vi "PIV_POD.vi"(0 "Data Folder":path=path "T:/Ensight_Data/NACA0015/NACA0015_NM_B/Test_A", 1 "PIV Meas Plane":enum16{"XY", "YZ", "XZ"}(ring)=enum."XZ", 2 "Row number":i32=1, 5 "Output Directory":path=path "T:/Ensight_Data/NACA0015/NACA0015_NM_B", 7 "XYZ Translation":dbl[](array[numeric])=[200.0, 8.0, -30.0], 9 "Case Name":string="Test_A_Case", 11 "PIV Freq (Hz)":dbl=7.25, 12 "Invert U":bool=TRUE, 13 "Invert V":bool) -> (4 "Progress Bar":i32(slide) scale=0.0..100.0, 6 "Status":string, 10 "# total vectors":i32=9858)   [LabVIEW 2022 SP3]
uses:
  <vilib>/Analysis/NI_AALBase.lvlib
  <vilib>/Analysis/1siggen.llb/Ramp Pattern by Samples.vi
  <vilib>/Utility/error.llb/DialogType.ctl
  <vilib>/Analysis/Matrix/NI_Matrix.lvlib
  <vilib>/Analysis/Matrix/Numeric/Multiply/Multiply - RM,RM.vi
  <vilib>/Analysis/NI_AALPro.lvlib
  <vilib>/Analysis/7linalg.llb/Real Eigenvalues and Vectors.vi
  <vilib>/Analysis/Matrix/Numeric/Conversions/Matrix To Array - CM.vi
  <vilib>/Analysis/Matrix/Numeric/Conversions/Array To Matrix - RA.vi
  <vilib>/Analysis/Matrix/Numeric/Conversions/Matrix To Array - RM.vi
  <vilib>/Analysis/Matrix/Numeric/Conversions/Array To Matrix - RA2.vi
panel:
  in  "Spot Data Cluster":T1
  out "u(Spot,mode)":dbl[][](array[numeric])
  out "v(Spot,mode)":dbl[][](array[numeric])
  out "Modal Energy":dbl[](array[numeric])
  out "eVal":dbl[](array[numeric]) format="%.2f"
  out "eVec":dbl[][](array[numeric])
  out "Uall(Spot,time)":dbl[][](array[numeric])
  out "v'(Spot,time)":dbl[][](array[numeric])
  out "u'(Spot,time)":dbl[][](array[numeric])
  out "Data Array (spot,Var)":dbl[][](array[numeric])
  out "File Paths":path[](array[path])
  out "Position Array (XYZ,spot)":dbl[][](array[numeric])
  out "Variable Names":string[](array[string])=["Record_Length", "CHC", "u_ms", "v_ms", "time_s", "Vel_mag_ms", "Turb_Stats_U_ms", "Turb_Stats_u2_m2s2", "Turb_Stats_u3_m3s3", "Turb_Stats_u4_m4s4", "Turb_Stats_TurbU_%", "Turb_Stats_Skew_u", "Turb_Stats_Kurt_u", "Turb_Stats_V_ms", "Turb_Stats_v2_m2s2", "Turb_Stats_v3_m3s3", "Turb_Stats_v4_m4s4", "Turb_Stats_TurbV_%", "Turb_Stats_Skew_v", "Turb_Stats_Kurt_v", "Turb_Stats_u2v2_m4s4", "Turb_Stats_uv3_m4s4", "Turb_Stats_u3v_m4s4", "Turb_Stats_uv2_m3s3", "Turb_Stats_u2v_m3s3", "Turb_Stats_uv_cc", "Turb_Stats_uv", "Turb_Stats_TKE_J", "Turb_Stats_Error_U_ms", "Turb_Stats_Error_u2_m2s2", "Turb_Stats_Error_u3_m3s3", "Turb_Stats_Error_u4_m4s4", "Turb_Stats_Error_TurbU_%", "Turb_Stats_Error_Skew_u", "Turb_Stats_Error_Kurt_u", "Turb_Stats_Error_V_ms", "Turb_Stats_Error_v2_m2s2", "Turb_Stats_Error_v3_m3s3", "Turb_Stats_Error_v4_m4s4", "Turb_Stats_Error_TurbV_%", "Turb_Stats_Error_Skew_v", "Turb_Stats_Error_Kurt_v", "Turb_Stats_Error_u2v2_m4s4", "Turb_Stats_Error_uv3_m4s4", "Turb_Stats_Error_u3v_m4s4", "Turb_Stats_Error_uv2_m3s3", "Turb_Stats_Error_u2v_m3s3", "Turb_Stats_Error_uv_cc", "Turb_Stats_Error_uv", "Turb_Stats_Error_TKE_J"]
  out "time s":dbl[](array[numeric])=[0.0, 0.20689655172413793, 0.41379310344827586]
  out "File Array":path[](array[path])=[path "T:/Ensight_Data/NACA0015/NACA0015_NM_A/Test_A_Trans/New folder/Test_A000000.T076.D000.P000.H000.L.vec", path "T:/Ensight_Data/NACA0015/NACA0015_NM_A/Test_A_Trans/New folder/Test_A000001.T076.D000.P000.H000.L.vec", path "T:/Ensight_Data/NACA0015/NACA0015_NM_A/Test_A_Trans/New folder/Test_A000002.T076.D000.P000.H000.L.vec"]
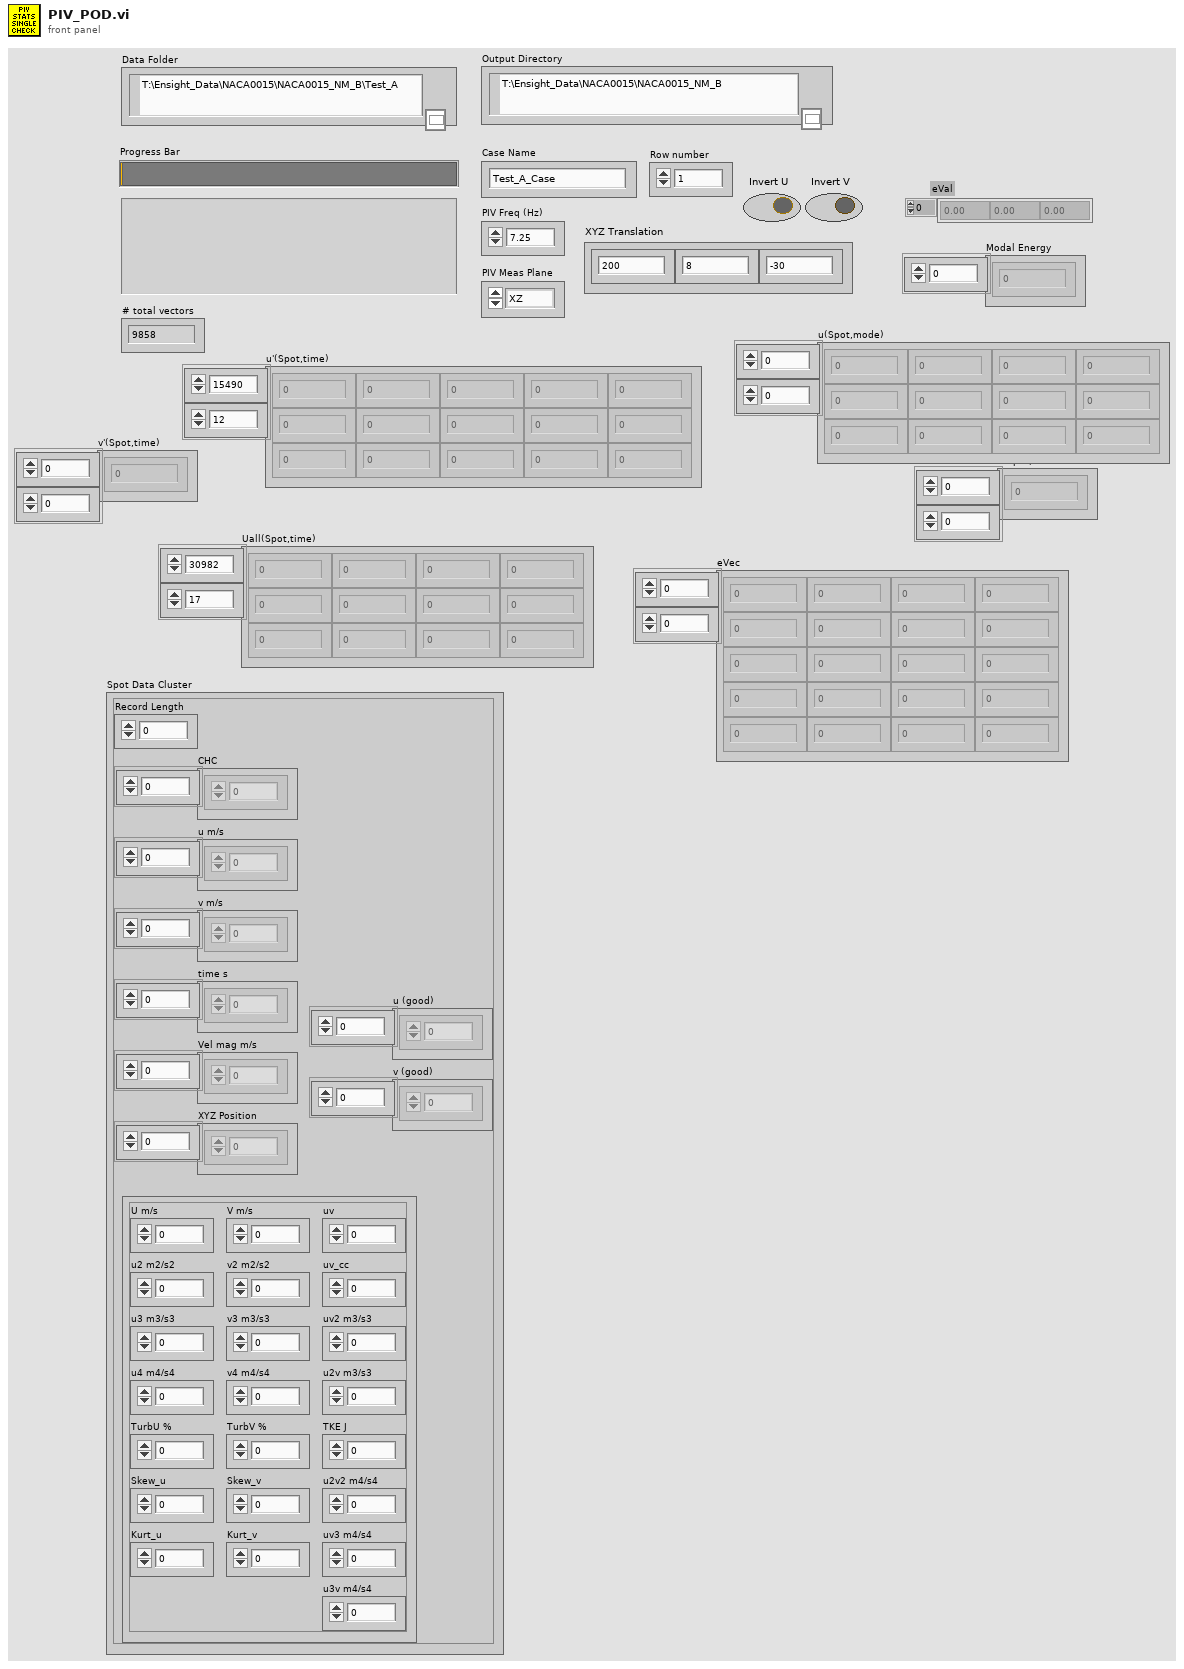
[diagram p1: front panel]
types:
  T1 = cluster{"Record Length":dbl, "CHC":dbl[], "u m/s":dbl[], "v m/s":dbl[], "time s":dbl[], "Vel mag m/s":dbl[], "XYZ Position":dbl[], "Turbulence Statistics":cluster{"U m/s":dbl, "u2 m2/s2":dbl, "u3 m3/s3":dbl, "u4 m4/s4":dbl, "TurbU %":dbl, "Skew_u":dbl, "Kurt_u":dbl, "V m/s":dbl, "v2 m2/s2":dbl, "v3 m3/s3":dbl, "v4 m4/s4":dbl, "TurbV %":dbl, "Skew_v":dbl, "Kurt_v":dbl, "u2v2 m4/s4":dbl, "uv3 m4/s4":dbl, "u3v m4/s4":dbl, "uv2 m3/s3":dbl, "u2v m3/s3":dbl, "uv_cc":dbl, "uv":dbl, "TKE J":dbl}, "v (good)":dbl[], "u (good)":dbl[]}
  T2 = cluster{"Record Length":dbl, "CHC":dbl[], "u m/s":dbl[], "v m/s":dbl[], "time s":dbl[], "Vel mag m/s":dbl[], "XYZ Position":dbl[], "Turbulence Statistics":cluster{"U m/s":dbl, "u2 m2/s2":dbl, "u3 m3/s3":dbl, "u4 m4/s4":dbl, "TurbU %":dbl, "Skew_u":dbl, "Kurt_u":dbl, "V m/s":dbl, "v2 m2/s2":dbl, "v3 m3/s3":dbl, "v4 m4/s4":dbl, "TurbV %":dbl, "Skew_v":dbl, "Kurt_v":dbl, "u2v2 m4/s4":dbl, "uv3 m4/s4":dbl, "u3v m4/s4":dbl, "uv2 m3/s3":dbl, "u2v m3/s3":dbl, "uv_cc":dbl, "uv":dbl, "TKE J":dbl}, "v (good)":dbl[], "u (good)":dbl[]}[]
  T3 = cluster{"Record Length":dbl, "CHC":dbl[], "u m/s":dbl[], "v m/s":dbl[], "time s":dbl[], "Vel mag m/s":dbl[], "XYZ Position":dbl[], " Turb Stats":cluster{"U m/s":dbl, "u2 m2/s2":dbl, "u3 m3/s3":dbl, "u4 m4/s4":dbl, "TurbU %":dbl, "Skew_u":dbl, "Kurt_u":dbl, "V m/s":dbl, "v2 m2/s2":dbl, "v3 m3/s3":dbl, "v4 m4/s4":dbl, "TurbV %":dbl, "Skew_v":dbl, "Kurt_v":dbl, "u2v2 m4/s4":dbl, "uv3 m4/s4":dbl, "u3v m4/s4":dbl, "uv2 m3/s3":dbl, "u2v m3/s3":dbl, "uv_cc":dbl, "uv":dbl, "TKE J":dbl}[], "Turb Stats Error":cluster{"U m/s":dbl, "u2 m2/s2":dbl, "u3 m3/s3":dbl, "u4 m4/s4":dbl, "TurbU %":dbl, "Skew_u":dbl, "Kurt_u":dbl, "V m/s":dbl, "v2 m2/s2":dbl, "v3 m3/s3":dbl, "v4 m4/s4":dbl, "TurbV %":dbl, "Skew_v":dbl, "Kurt_v":dbl, "u2v2 m4/s4":dbl, "uv3 m4/s4":dbl, "u3v m4/s4":dbl, "uv2 m3/s3":dbl, "u2v m3/s3":dbl, "uv_cc":dbl, "uv":dbl, "TKE J":dbl}[], "u (good)":dbl[], "v (good)":dbl[]}
  T4 = cluster{"U m/s":dbl, "u2 m2/s2":dbl, "u3 m3/s3":dbl, "u4 m4/s4":dbl, "TurbU %":dbl, "Skew_u":dbl, "Kurt_u":dbl, "V m/s":dbl, "v2 m2/s2":dbl, "v3 m3/s3":dbl, "v4 m4/s4":dbl, "TurbV %":dbl, "Skew_v":dbl, "Kurt_v":dbl, "u2v2 m4/s4":dbl, "uv3 m4/s4":dbl, "u3v m4/s4":dbl, "uv2 m3/s3":dbl, "u2v m3/s3":dbl, "uv_cc":dbl, "uv":dbl, "TKE J":dbl}
  T5 = cluster{"U m/s":dbl, "u2 m2/s2":dbl, "u3 m3/s3":dbl, "u4 m4/s4":dbl, "TurbU %":dbl, "Skew_u":dbl, "Kurt_u":dbl, "V m/s":dbl, "v2 m2/s2":dbl, "v3 m3/s3":dbl, "v4 m4/s4":dbl, "TurbV %":dbl, "Skew_v":dbl, "Kurt_v":dbl, "u2v2 m4/s4":dbl, "uv3 m4/s4":dbl, "u3v m4/s4":dbl, "uv2 m3/s3":dbl, "u2v m3/s3":dbl, "uv_cc":dbl, "uv":dbl, "TKE J":dbl}[]
  T6 = cluster{"Record Length":dbl, "CHC":dbl[], "u m/s":dbl[], "v m/s":dbl[], "time s":dbl[], "Vel mag m/s":dbl[], "XYZ Position":dbl[], " Turb Stats":cluster{"U m/s":dbl, "u2 m2/s2":dbl, "u3 m3/s3":dbl, "u4 m4/s4":dbl, "TurbU %":dbl, "Skew_u":dbl, "Kurt_u":dbl, "V m/s":dbl, "v2 m2/s2":dbl, "v3 m3/s3":dbl, "v4 m4/s4":dbl, "TurbV %":dbl, "Skew_v":dbl, "Kurt_v":dbl, "u2v2 m4/s4":dbl, "uv3 m4/s4":dbl, "u3v m4/s4":dbl, "uv2 m3/s3":dbl, "u2v m3/s3":dbl, "uv_cc":dbl, "uv":dbl, "TKE J":dbl}[], "Turb Stats Error":cluster{"U m/s":dbl, "u2 m2/s2":dbl, "u3 m3/s3":dbl, "u4 m4/s4":dbl, "TurbU %":dbl, "Skew_u":dbl, "Kurt_u":dbl, "V m/s":dbl, "v2 m2/s2":dbl, "v3 m3/s3":dbl, "v4 m4/s4":dbl, "TurbV %":dbl, "Skew_v":dbl, "Kurt_v":dbl, "u2v2 m4/s4":dbl, "uv3 m4/s4":dbl, "u3v m4/s4":dbl, "uv2 m3/s3":dbl, "u2v m3/s3":dbl, "uv_cc":dbl, "uv":dbl, "TKE J":dbl}[], "u (good)":dbl[], "v (good)":dbl[]}[]
  T7 = typedef "NI_Matrix.lvlib/RealMatrix.ctl" = dbl[][]
  T8 = typedef "NI_Matrix.lvlib/ComplexMatrix.ctl" = cdb[][]
  T9 = typedef "DialogType.ctl" = u16
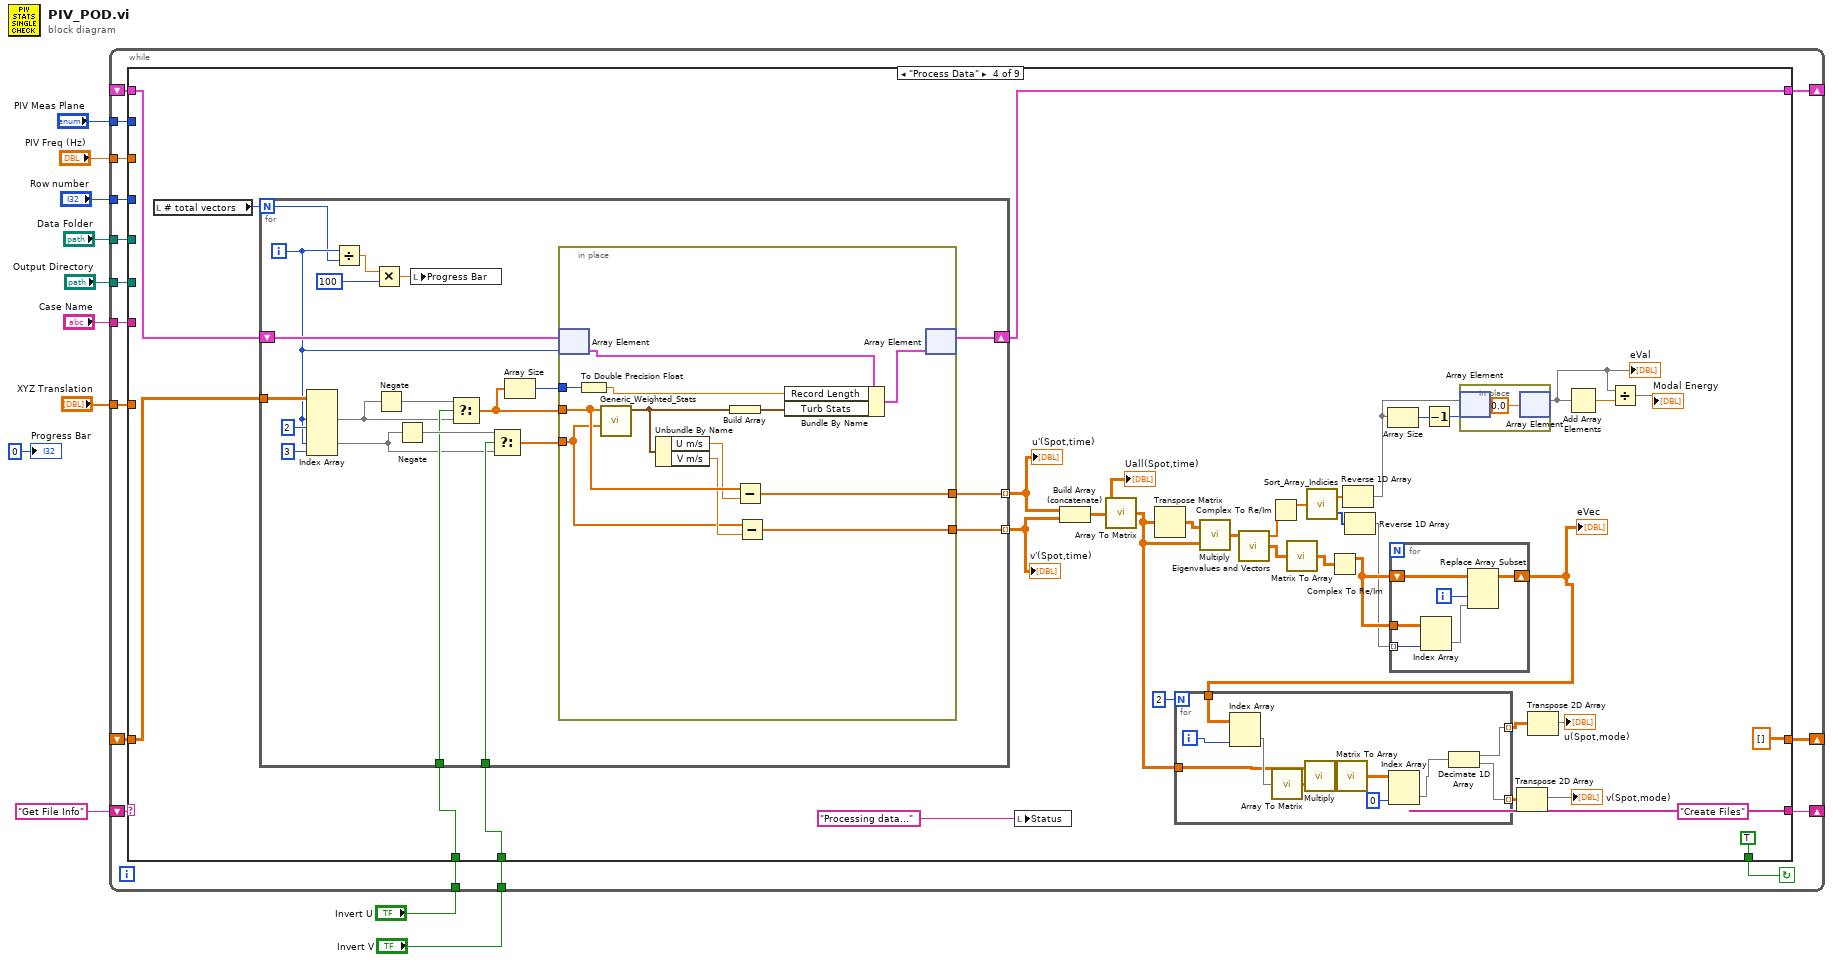
[diagram p0: block diagram]
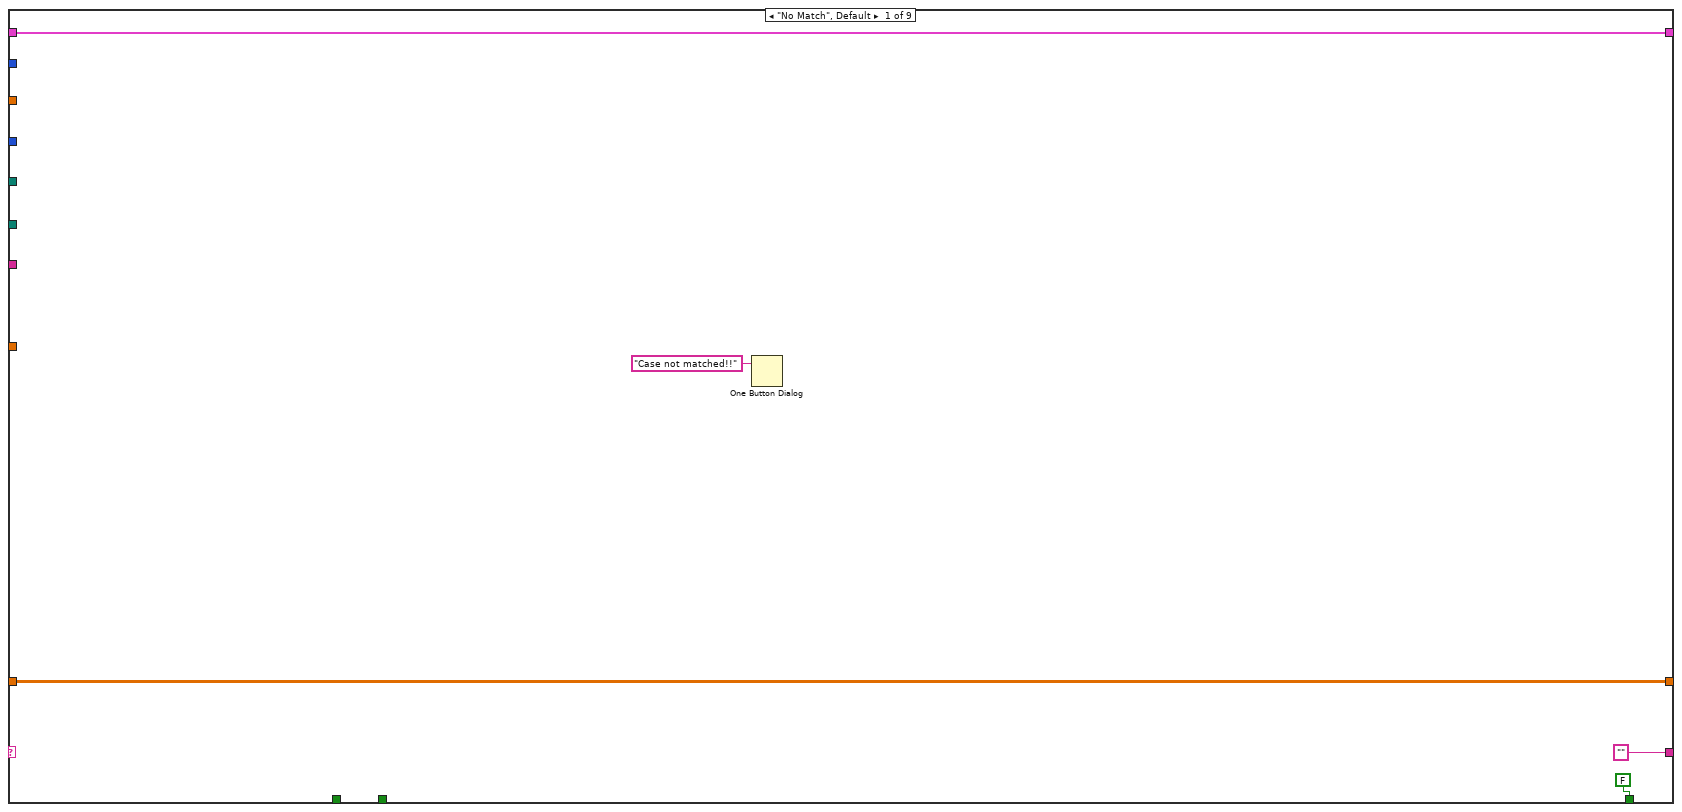
[diagram p2: hidden frame]
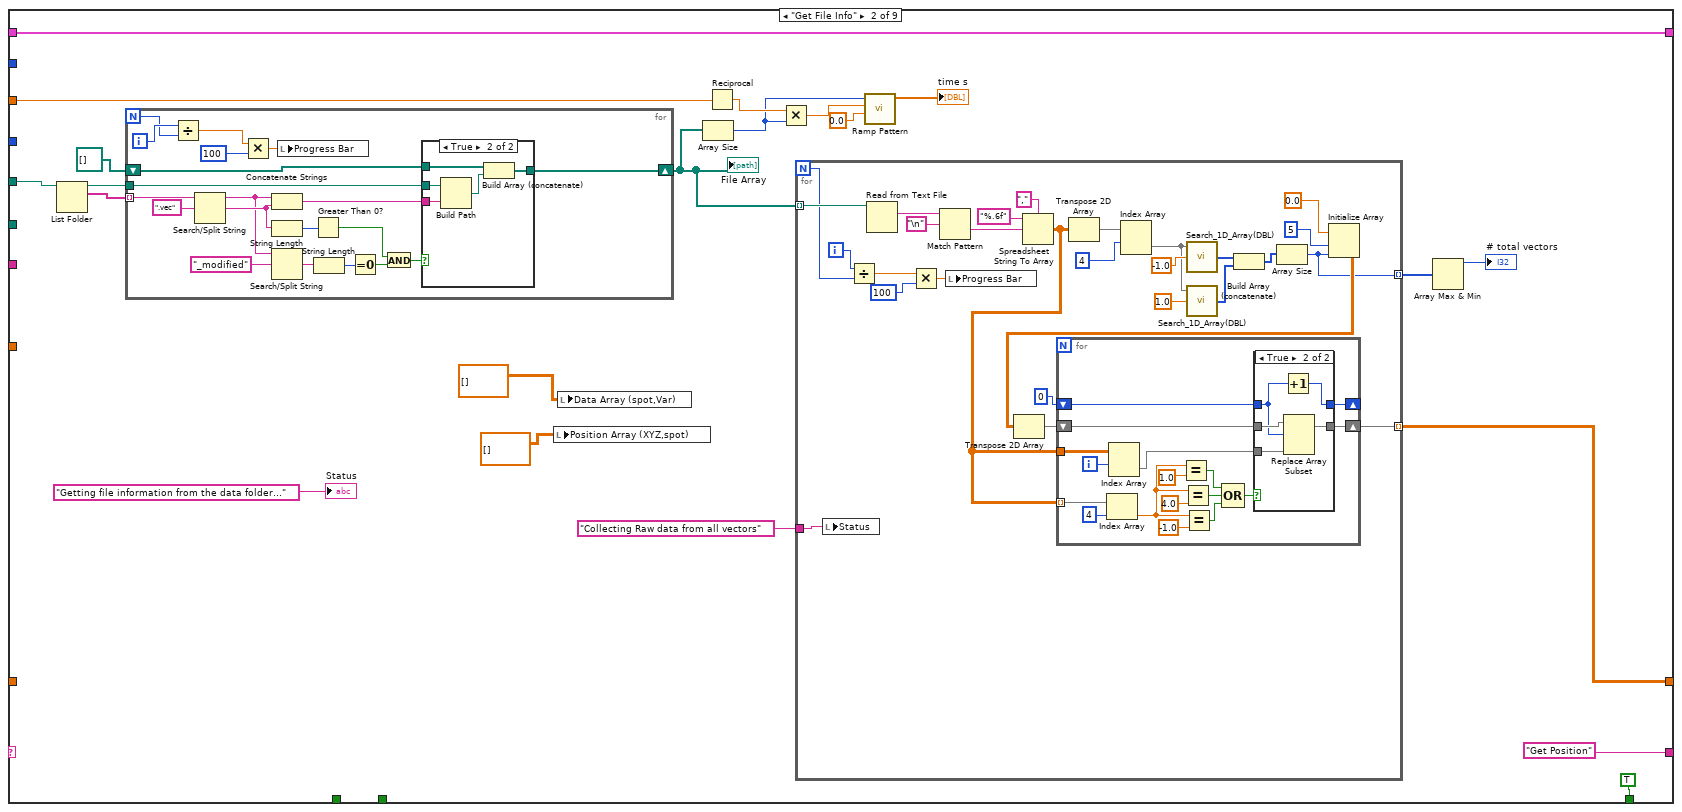
[diagram p3: hidden frame]
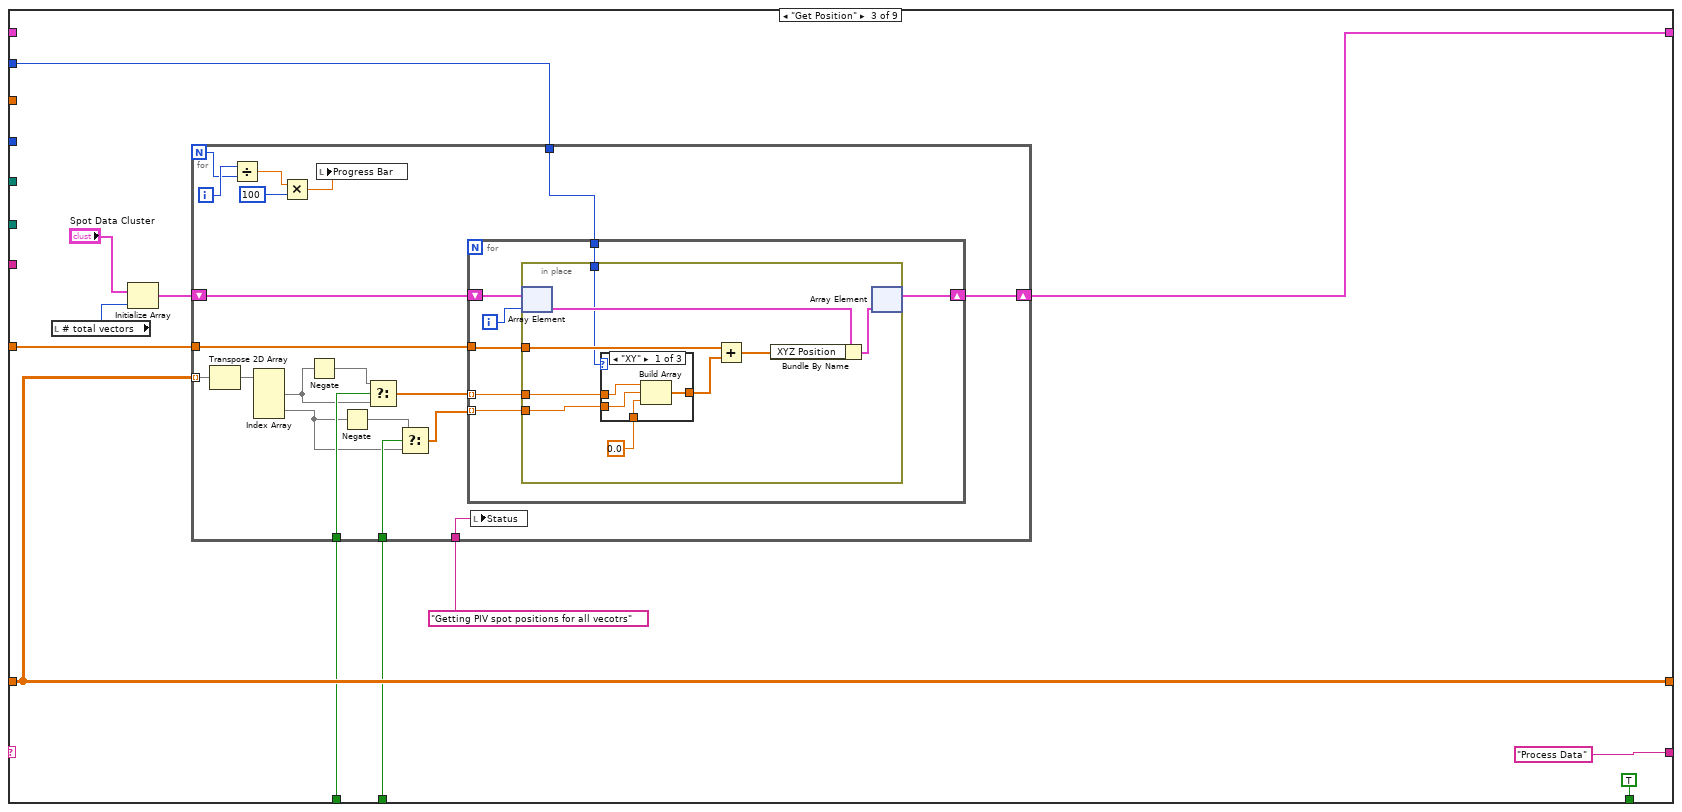
[diagram p6: hidden frame]
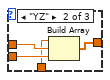
[diagram p7: hidden frame]
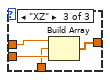
[diagram p8: hidden frame]
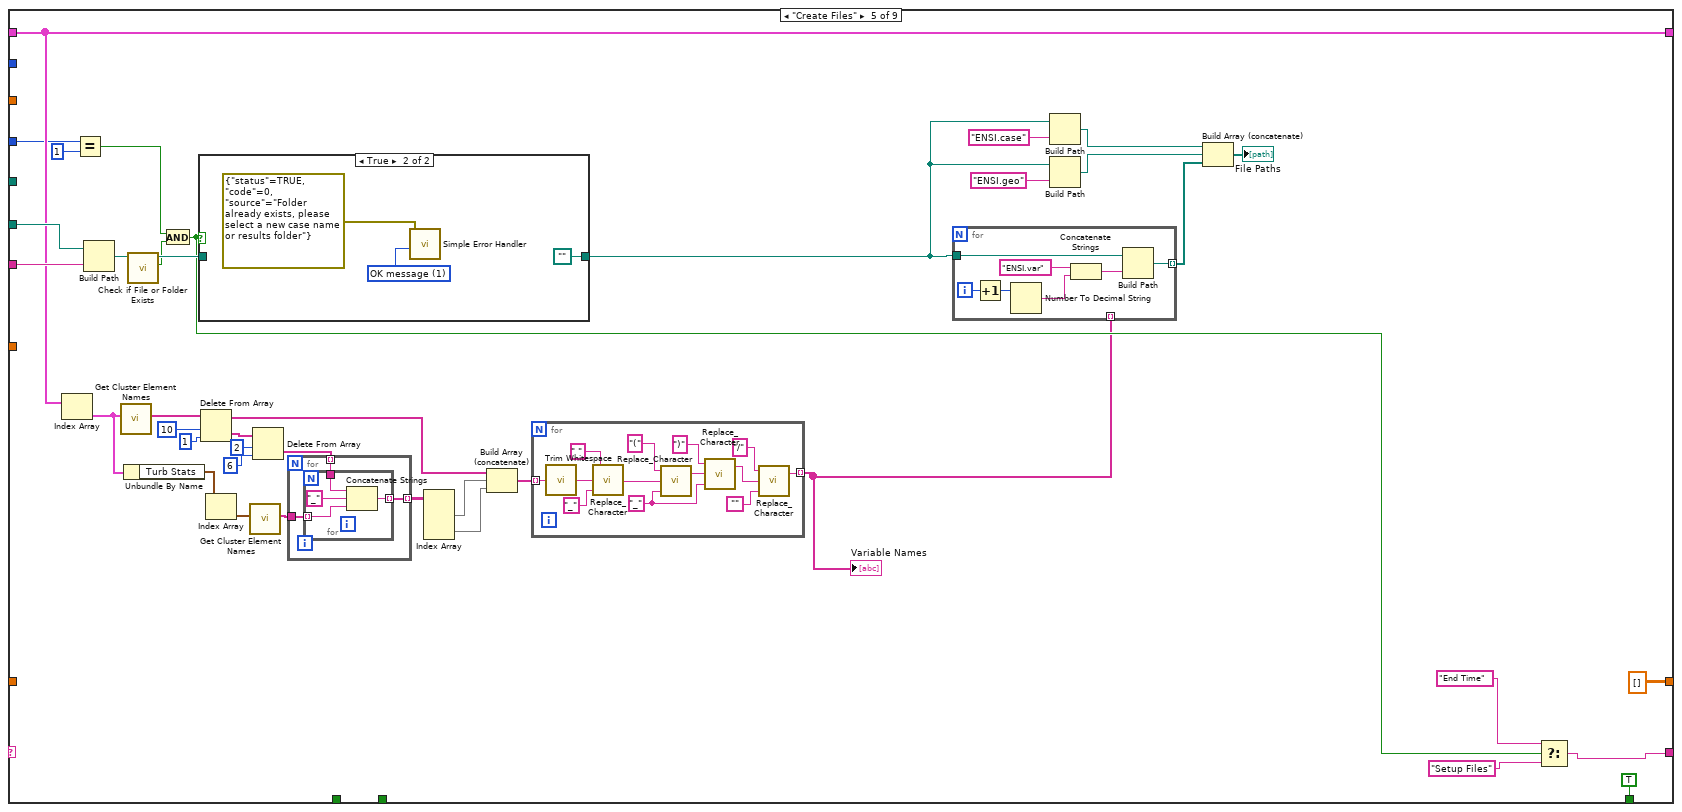
[diagram p9: hidden frame]
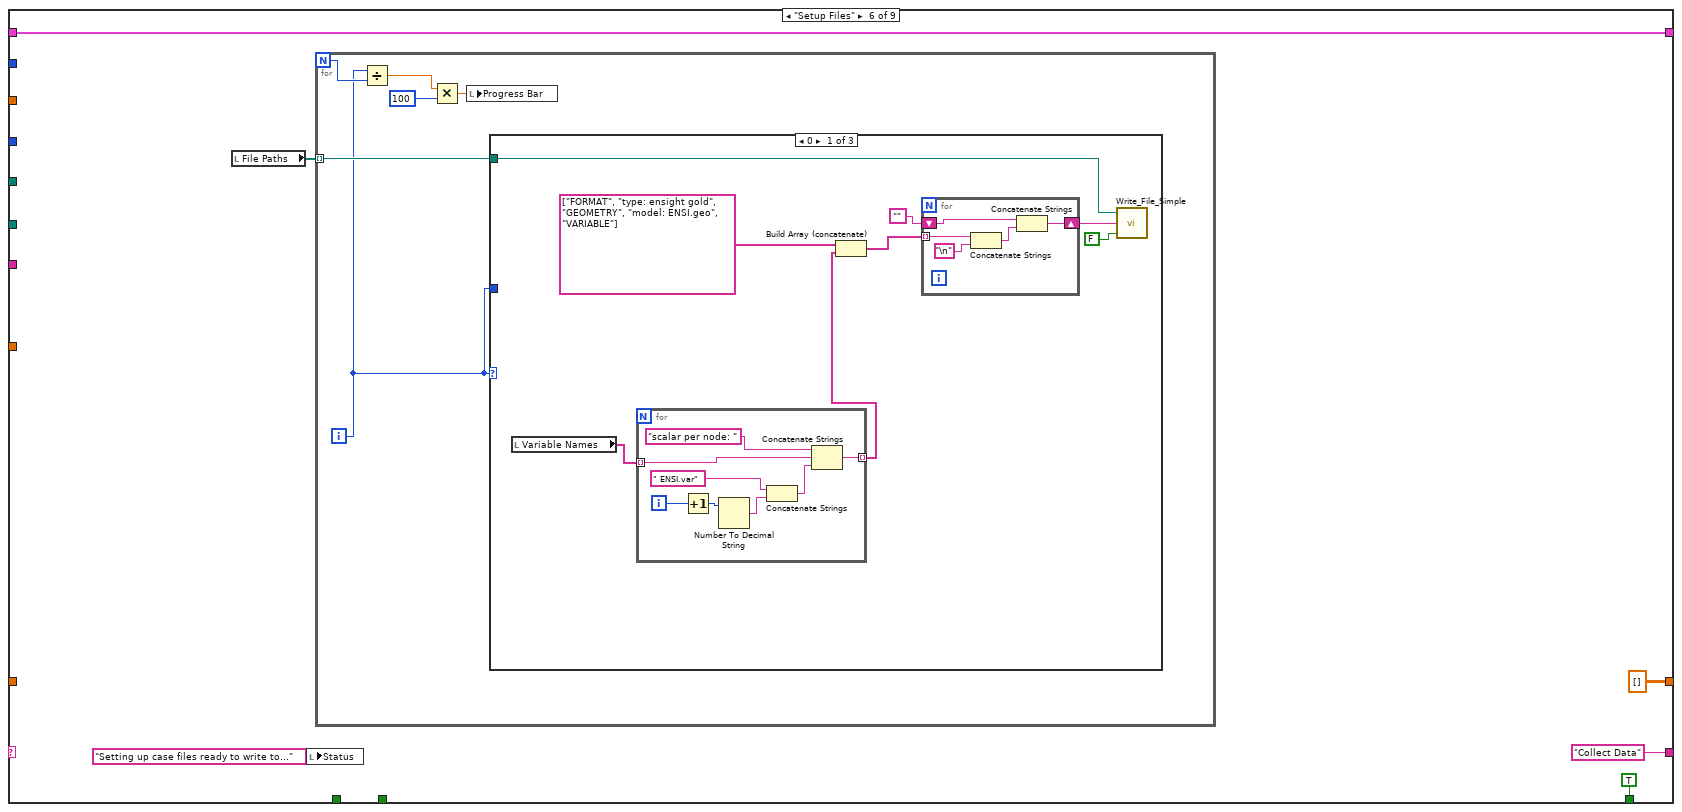
[diagram p11: hidden frame]
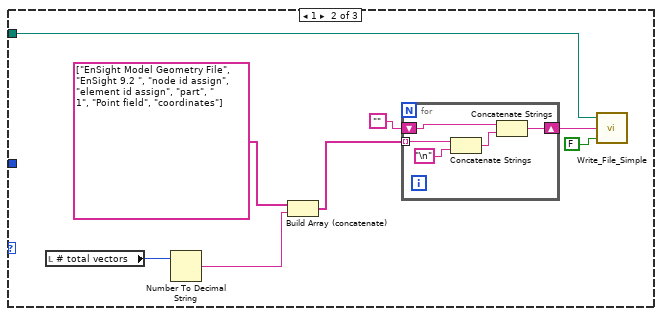
[diagram p12: hidden frame]
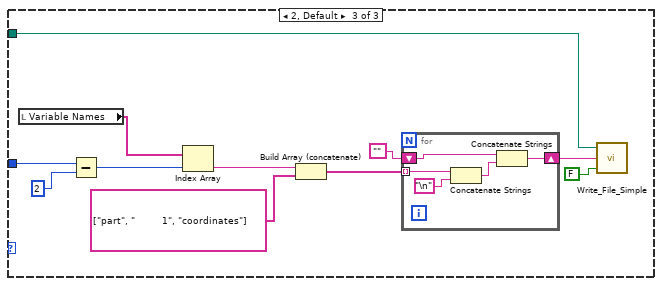
[diagram p13: hidden frame]
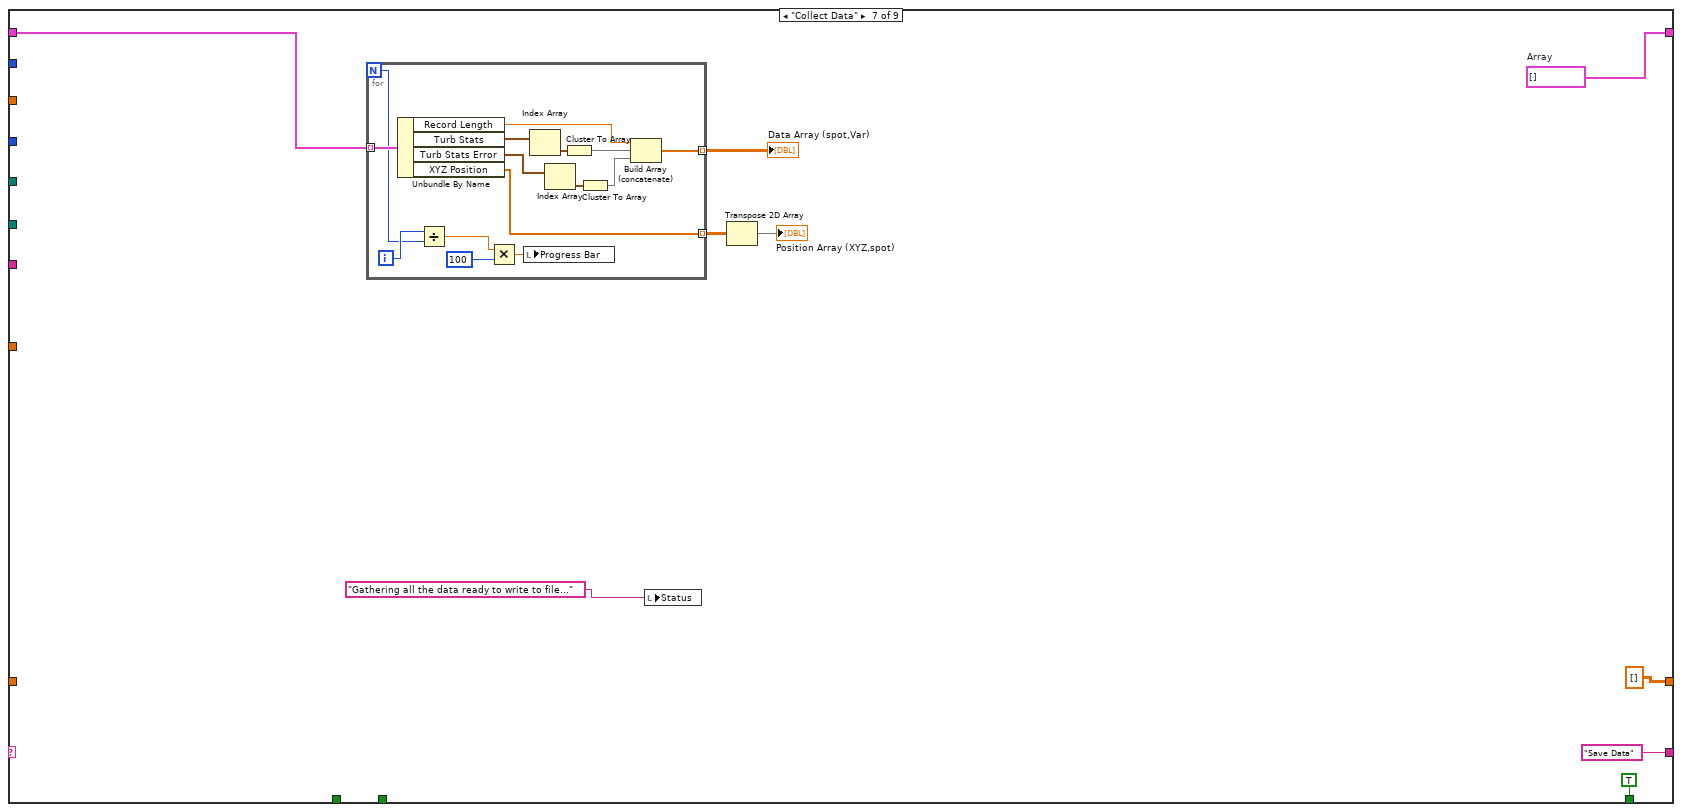
[diagram p14: hidden frame]
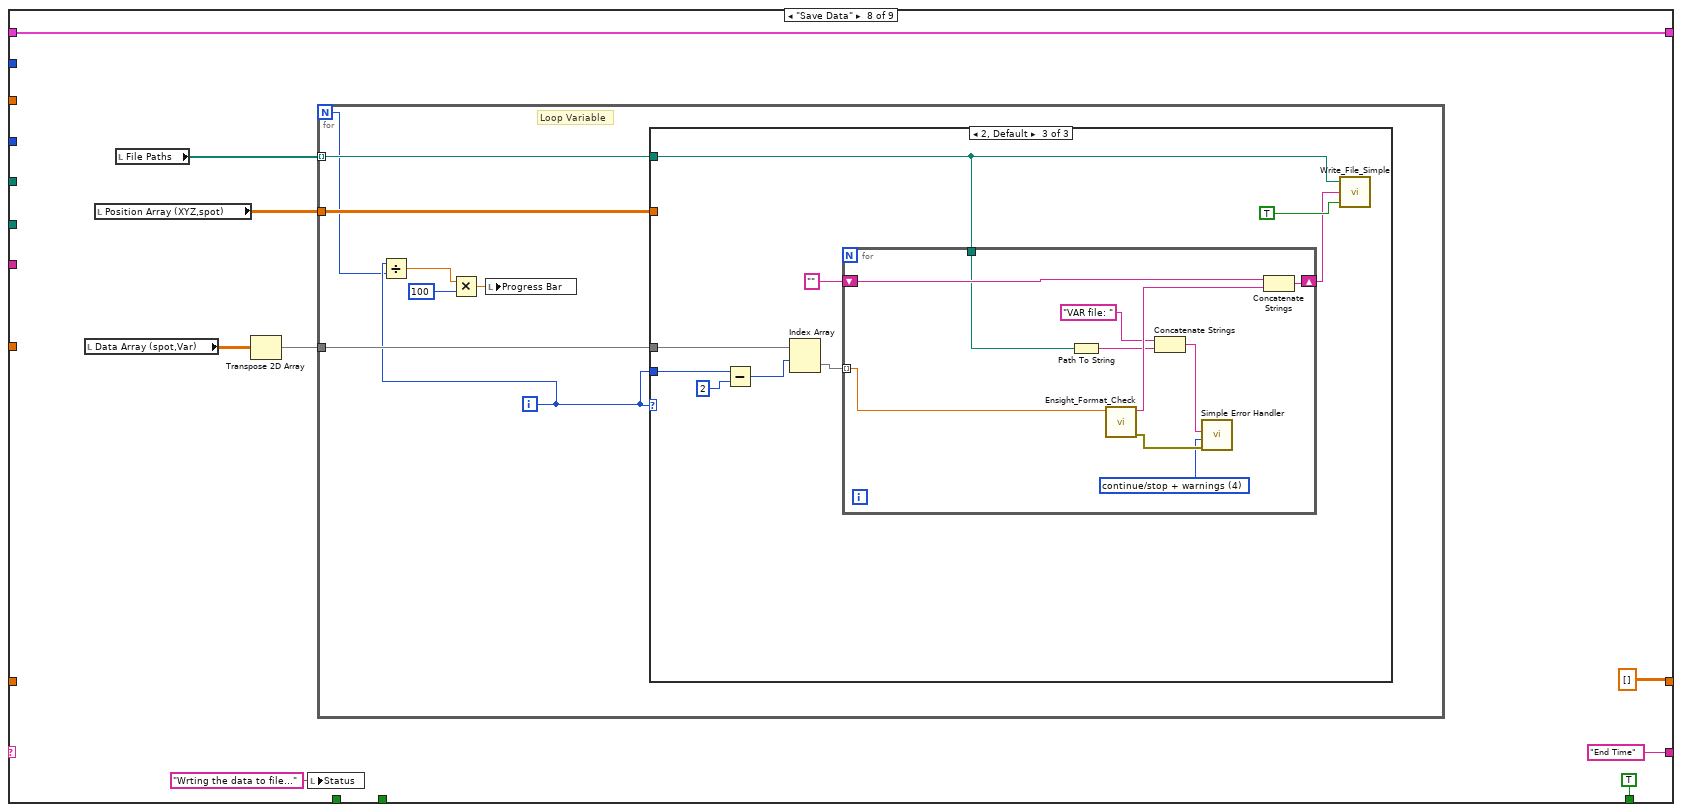
[diagram p15: hidden frame]
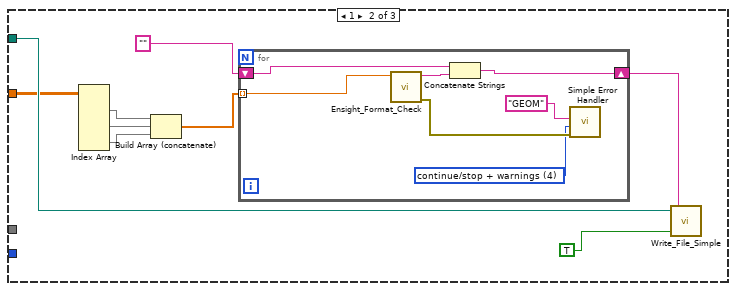
[diagram p17: hidden frame]
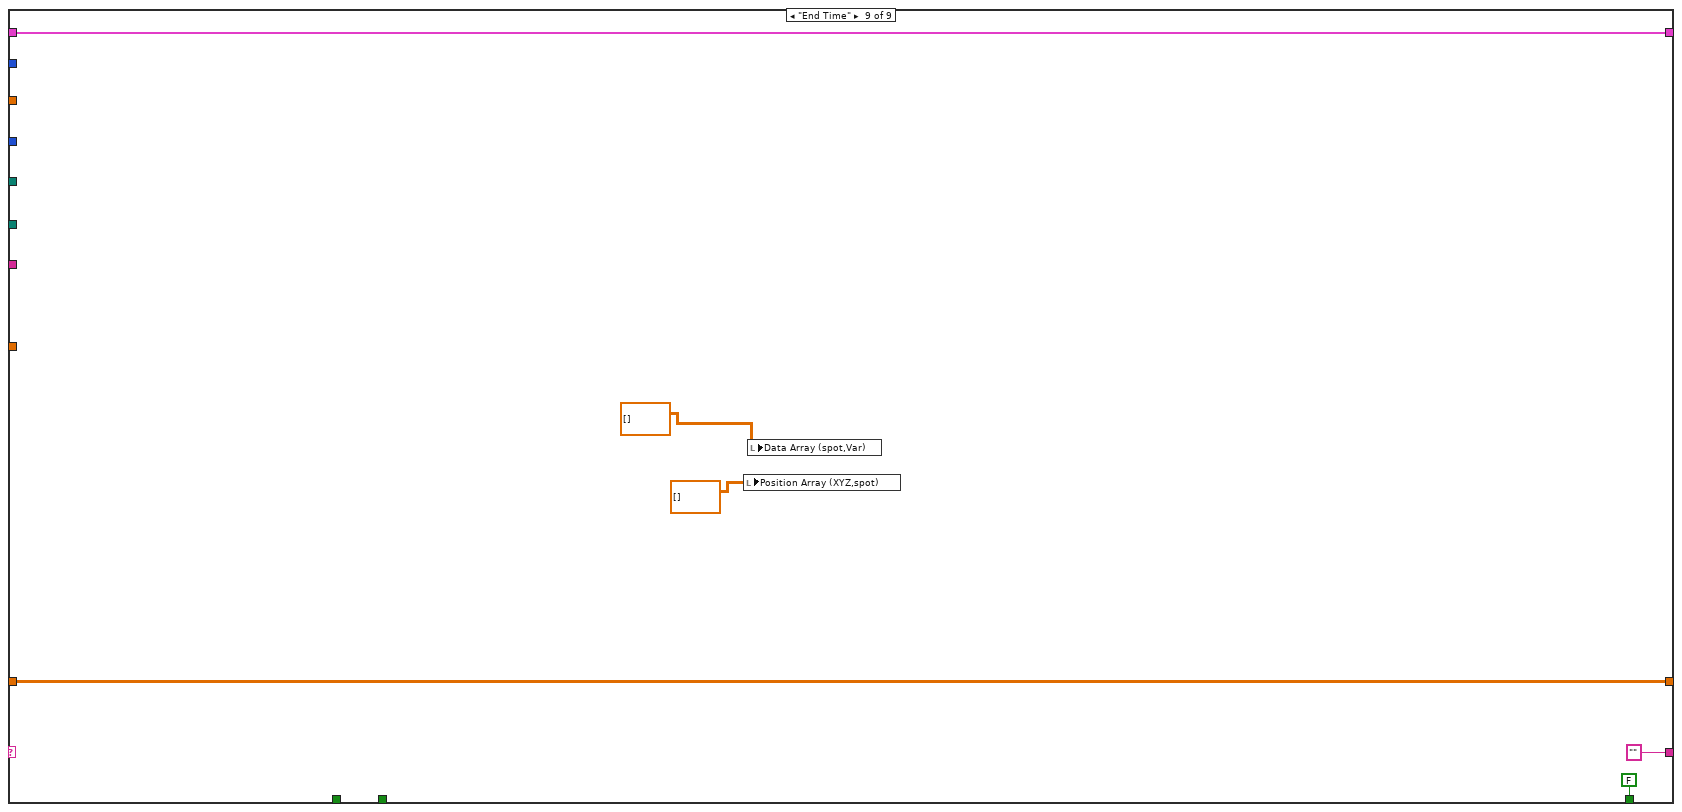
[diagram p18: hidden frame]
diagram:
  n1 = while {
    shift-right: [w26] -> _
    shift-left: "Get File Info" -> [w27]
    tunnel: "Data Folder" -> [w25]
    tunnel: "Output Directory" -> [w23]
    tunnel: "Case Name" -> [w22]
    tunnel: "PIV Freq (Hz)" -> [w21]
    tunnel: "PIV Meas Plane" -> [w20]
    tunnel: "XYZ Translation" -> [w19]
    shift-right: [w18] -> _
    shift-left: _ -> [w17]
    tunnel: "Row number" -> [w16]
    tunnel: "Invert V" -> [w15]
    tunnel: "Invert U" -> [w14]
    shift-right: [w13] -> _
    shift-left: _ -> [w12]
    stop <- w24 continue-if-true
    n2 = case shown="\"Process Data\"" w27 {
      tunnel: ["" "Get Position" "Process Data" "Create Files" w292 "Collect Data" ("t") "Save Data" ("t") "End Time" ("t") "" ("t")] -> w26
      tunnel: w25 -> [_ w48 _ _ _ _ _ _ _]
      tunnel: [FALSE TRUE TRUE TRUE TRUE TRUE TRUE TRUE FALSE] -> w24
      tunnel: w23 -> [_ _ _ _ w316 _ _ _ _]
      tunnel: w22 -> [_ _ _ _ w317 _ _ _ _]
      tunnel: w21 -> [_ w47 _ _ _ _ _ _ _]
      tunnel: w20 -> [_ _ w140 _ _ _ _ _ _]
      tunnel: w19 -> [_ _ w141 _ _ _ _ _ _]
      tunnel: [w30 w35 w135 w222 w302 w351 w415 w441 w488] -> w18
      tunnel: w17 -> [w30 w35 _ w226 w302 w351 w417 w441 w488]
      tunnel: w16 -> [_ _ _ _ w298 _ _ _ _]
      tunnel: w15 -> [_ _ w133 w223 _ _ _ _ _]
      tunnel: w14 -> [_ _ w132 w224 _ _ _ _ _]
      tunnel: [w28 w33 w134 dbl[][][] [] ("GoodRawData(time,spot)") dbl[][][] [] ("GoodRawData(time,spot)") dbl[][][] [] ("GoodRawData(time,spot)") dbl[][][] [] ("GoodRawData(time,spot)") dbl[][][] [] ("GoodRawData(time,spot)") w487] -> w13
      tunnel: w12 -> [w28 _ w134 w225 _ _ _ _ w487]
      frame "No Match", Default {
        n3 = One Button Dialog(message="Case not matched!!") -> ()  [unwired: 1 in, 1 out]
      }
      frame "Get File Info" {
        n4 = List Folder(path=w48) -> (path out=w50:path, filenames=w51:string[])  [unwired: 3 in, 2 out]
        n5 = for {
          N -> [w106]
          tunnel: w51 -> [w125] mode=indexing
          shift-right: [w118] -> w38
          shift-left: path[] [] -> [w120]
          tunnel: w50 -> [w119]
          i -> [w107]
          n6 = Divide(x=w107, y=w106) -> (x/y=w109:dbl)
          n7 = Search/Split String(string=w125, search string/char (-)=".vec") -> (substring before match=w116:string, match + rest of string=w122:string)  [unwired: 1 in, 1 out]
          n8 = Multiply(x=w109, y=100) -> (x*y=w110:dbl)
          n9 = Concatenate Strings(w116, w122) -> (w121:string)
          n10 = String Length(string=w122) -> (length=w123:i32)
          n11 = Search/Split String(string=w116, search string/char (-)="_modified") -> (match + rest of string=w114:string)  [unwired: 1 in, 2 out]
          n12 = local write "Progress Bar"(w110) -> ()
          n13 = Greater Than 0?(x=w123) -> (x > 0?=w117:bool)
          n14 = String Length(string=w114) -> (length=w113:i32)
          n15 = Equal To 0?(x=w113) -> (x = 0?=w112:bool)
          n16 = And(x=w117, y=w112) -> (x .and. y?=w111:bool)
          n17 = case shown="True" w111 {
            tunnel: w121 -> [_ w131]
            tunnel: w120 -> [w126 w127]
            tunnel: w119 -> [_ w130]
            tunnel: [w126 w128] -> w118
            frame False {
            }
            frame True {
              n18 = Build Path(base path=w130, name or relative path=w131) -> (appended path=w129:path)
              n19 = Build Array (concatenate)(w127, w129) -> (w128:path[])
            }
          }
        }
        "File Array" <- w38
        n20 = local write "Position Array (XYZ,spot)"(dbl[][] [] ("Position Array")) -> ()
        n21 = local write "Data Array (spot,Var)"(dbl[][] [] ("Data Array")) -> ()
        n22 = Array Size(array=w38) -> (size(s)=w42:i32)
        n23 = Reciprocal(x=w47) -> (1/x=w45:dbl)
        n24 = Multiply(x=w45, y=w42) -> (x*y=w46:dbl)
        n25 = for {
          N -> [w65]
          tunnel: w38 -> [w72] mode=indexing
          tunnel: [w54] -> w37 mode=indexing
          tunnel: [w69] -> w33 mode=indexing
          tunnel: "Collecting Raw data from all vectors" ("Status") -> [w63]
          i -> [w64]
          n26 = local write "Status"(w63) -> ()
          n27 = Divide(x=w64, y=w65) -> (x/y=w67:dbl)
          n28 = Read from Text File(file (use dialog)=w72) -> (text=w81:string)  [unwired: 3 in, 3 out]
          n29 = Multiply(x=w67, y=100) -> (x*y=w66:dbl)
          n30 = Match Pattern(string=w81, regular expression="\n") -> (after substring=w77:string)  [unwired: 1 in, 3 out]
          n31 = local write "Progress Bar"(w66) -> ()
          n32 = Spreadsheet String To Array(delimiter (Tab)=",", format string="%.6f", spreadsheet string=w77) -> (array=w60:dbl[][])  [unwired: 1 in]
          n33 = Transpose 2D Array(2D array=w60) -> (transposed array=w76:dbl[][])
          n34 = Index Array(array=w76, index (row)=4) -> (element=w59:dbl[])  [unwired: 1 in]
          n35 = call "Search_1D_Array(DBL).vi"("Array"=w59, "Element Data"=-1.0) -> ("Indicies of Elements"=w58:i32[])  [unwired: 6 in, 1 out]
          n36 = call "Search_1D_Array(DBL).vi"("Array"=w59, "Element Data"=1.0) -> ("Indicies of Elements"=w56:i32[])  [unwired: 6 in, 1 out]
          n37 = Build Array (concatenate)(w58, w56) -> (w57:i32[])
          n38 = Array Size(array=w57) -> (size(s)=w54:i32)
          n39 = Initialize Array(0.0 ("element"), 5 ("dimension size"), w54) -> (w70:dbl[][])
          n40 = Transpose 2D Array(2D array=w70) -> (transposed array=w71:dbl[][])
          n41 = for {
            tunnel: w60 -> [w93] mode=indexing
            shift-right: [w96] -> w69
            shift-left: w71 -> [w91]
            shift-right: [w95] -> _
            shift-left: 0 ("y") -> [w94]
            tunnel: w60 -> [w92]
            i -> [w90]
            n42 = Index Array(array=w93, index=4) -> (element=w87:dbl)
            n43 = Index Array(array=w92, index (row)=w90) -> (element=w97:dbl[])  [unwired: 1 in]
            n44 = Equal?(x=w87, y=1.0) -> (x = y?=w83:bool)
            n45 = Equal?(x=w87, y=4.0) -> (x = y?=w84:bool)
            n46 = Equal?(x=w87, y=-1.0) -> (x = y?=w85:bool)
            n47 = Compound Arithmetic op=OR(w83, w84, w85) -> (w82:bool)
            n48 = case shown="True" w82 {
              tunnel: w97 -> [_ w103]
              tunnel: w91 -> [w100 w105]
              tunnel: [w100 w104] -> w96
              tunnel: [w99 w102] -> w95
              tunnel: w94 -> [w99 w101]
              frame False {
              }
              frame True {
                n49 = Increment(x=w101) -> (x+1=w102:i32)
                n50 = Replace Array Subset(array=w105, new element=w103, index (row)=w101) -> (w104:dbl[][])  [unwired: 1 in]
              }
            }
          }
        }
        n51 = call-poly <vilib>:"Ramp Pattern.vi"("start"=0.0, "end"=w46, "samples"=w42) -> ("Ramp Pattern"=→"time s":dbl[])  [unwired: 7 in, 1 out]
        n52 = Array Max & Min(array=w37) -> (max value=→"# total vectors":i32)  [unwired: 3 out]
        "Status" <- "Getting file information from the data folder..." ("Status")
      }
      frame "Get Position" {
        n53 = local read "# total vectors"() -> (w139:i32)
        n54 = Initialize Array("Spot Data Cluster", w139) -> (w137:T2)
        n55 = for {
          N -> [w156]
          shift-right: [w161] -> w135
          shift-left: w137 -> [w162]
          tunnel: w134 -> [w154] mode=indexing
          tunnel: w141 -> [w163]
          tunnel: w140 -> [w155]
          tunnel: "Getting PIV spot positions for all vecotrs" ("Status") -> [w152]
          tunnel: w133 -> [w151]
          tunnel: w132 -> [w150]
          i -> [w157]
          n56 = Transpose 2D Array(2D array=w154) -> (transposed array=w153:dbl[][])
          n57 = Divide(x=w157, y=w156) -> (x/y=w159:dbl)
          n58 = Index Array(array=w153) -> (element #1=w146:dbl[], element #2=w144:dbl[])  [unwired: 4 in]
          n59 = Multiply(x=w159, y=100) -> (x*y=w160:dbl)
          n60 = Negate(x=w146) -> (-x=w147:dbl[])
          n61 = local write "Progress Bar"(w160) -> ()
          n62 = Negate(x=w144) -> (-x=w145:dbl[])
          n63 = Select(t=w147, s=w150, f=w146) -> (s? t:f=w148:dbl[])
          n64 = Select(t=w145, s=w151, f=w144) -> (s? t:f=w149:dbl[])
          n65 = for {
            tunnel: w148 -> [w170] mode=indexing
            tunnel: w149 -> [w169] mode=indexing
            tunnel: w163 -> [w168]
            shift-right: [w165] -> w161
            shift-left: w162 -> [w167]
            tunnel: w155 -> [w164]
            i -> [w166]
            n66 = in-place {
              in-place-border: w170 -> [w177]
              in-place-border: w169 -> [w176]
              in-place-border: w168 -> [w175]
              in-place-border: w164 -> [w171]
              n67 = in-place-array #1(w167, w166) -> (w174:T1)
              n68 = case shown="\"XY\"" w171 {
                tunnel: w177 -> [w181 w187 w191]
                tunnel: w176 -> [w182 w186 w190]
                tunnel: 0.0 ("element") -> [w183 w185 w189]
                tunnel: [w180 w184 w188] -> w179
                frame "XY" {
                  n69 = Build Array(w181, w182, w183) -> (w180:dbl[])
                }
                frame "YZ" {
                  n70 = Build Array(w185, w187, w186) -> (w184:dbl[])
                }
                frame "XZ" {
                  n71 = Build Array(w191, w189, w190) -> (w188:dbl[])
                }
              }
              n72 = Add(x=w175, y=w179) -> (x+y=w173:dbl[])
              n73 = Bundle By Name(cluster=w174, "XYZ Position"=w173) -> (w172:T1)
              n74 = in-place-array #1(w172) -> (w165:T2)  [unwired: 1 out]
            }
          }
          n75 = local write "Status"(w152) -> ()
        }
      }
      frame "Process Data" {
        n76 = local read "# total vectors"() -> (w227:i32)
        n77 = for {
          N: w227 -> [w251]
          tunnel: w223 -> [w261]
          tunnel: w224 -> [w260]
          tunnel: w225 -> [w255]
          shift-right: [w254] -> w222
          shift-left: w226 -> [w253]
          tunnel: [w247] -> w217 mode=indexing
          tunnel: [w246] -> w216 mode=indexing
          i -> [w252]
          n78 = Index Array(array=w255, index (dim 1) #1=w252, index (dim 2) #1=2 ("disabled index (col)"), index (dim 1) #2=w252, index (dim 2) #2=3 ("disabled index (col)")) -> (element #1=w257:dbl[], element #2=w256:dbl[])  [unwired: 2 in]
          n79 = Divide(x=w252, y=w251) -> (x/y=w263:dbl)
          n80 = Multiply(x=w263, y=100) -> (x*y=w264:dbl)
          n81 = Negate(x=w257) -> (-x=w266:dbl[])
          n82 = Negate(x=w256) -> (-x=w265:dbl[])
          n83 = local write "Progress Bar"(w264) -> ()
          n84 = Select(t=w266, s=w260, f=w257) -> (s? t:f=w249:dbl[])
          n85 = Select(t=w265, s=w261, f=w256) -> (s? t:f=w248:dbl[])
          n86 = Array Size(array=w249) -> (size(s)=w250:i32)
          n87 = in-place {
            in-place-border: w249 -> [w272]
            in-place-border: w248 -> [w269]
            in-place-border: w250 -> [w274]
            in-place-border: [w268] -> w247
            in-place-border: [w267] -> w246
            n88 = in-place-array #2(w253, w252) -> (w278:T3)
            n89 = To Double Precision Float(number=w274) -> (double precision float=w276:dbl)
            n90 = call "Generic_Weighted_Stats.vi"("v"=w269, "u"=w272) -> ("Turbulence Statistics"=w273:T4)  [unwired: 9 in]
            n91 = Unbundle By Name(w273) -> ("U m/s"=w271:dbl, "V m/s"=w270:dbl)
            n92 = Build Array(w273) -> (w275:T5)
            n93 = Subtract(x=w272, y=w271) -> (x-y=w268:dbl[])
            n94 = Subtract(x=w269, y=w270) -> (x-y=w267:dbl[])
            n95 = Bundle By Name(cluster=w278, "Record Length"=w276, "Turb Stats"=w275) -> (w277:T3)
            n96 = in-place-array #2(w277) -> (w254:T6)  [unwired: 1 out]
          }
        }
        "u'(Spot,time)" <- w217
        "v'(Spot,time)" <- w216
        n97 = local write "Status"("Processing data..." ("Status")) -> ()
        n98 = Build Array (concatenate)(w217, w216) -> (w215:dbl[][])
        "Uall(Spot,time)" <- w215
        n99 = call-poly <vilib>:"Array To Matrix.vi"("Real 2D Array"=w215) -> ("Real Matrix"=w200:T7)
        n100 = Transpose Matrix(1:w200) -> (0:w214:T7)
        n101 = call-poly <vilib>:"Multiply.vi"("Real Matrix B"=w200, "Real Matrix A"=w214) -> ("A * B"=w211:T7)
        n102 = call-poly <vilib>:"Eigenvalues and Vectors.vi"("Input Matrix"=w211) -> ("Eigenvectors"=w213:T8, "Eigenvalues"=w212:cdb[])  [unwired: 2 in, 1 out]
        n103 = Complex To Re/Im(x + iy=w212) -> (x=w209:dbl[])  [unwired: 1 out]
        n104 = call-poly <vilib>:"Matrix To Array.vi"("Complex Matrix"=w213) -> ("Complex 2D Array"=w210:cdb[][])
        n105 = call "Sort_Array_Indicies.vi"("unsorted array"=w209) -> ("sorted array"=w205:dbl[], "Sort Index"=w208:i32[])
        n106 = Complex To Re/Im(x + iy=w210) -> (x=w207:dbl[][])  [unwired: 1 out]
        n107 = Reverse 1D Array(array=w205) -> (reversed array=w195:dbl[])
        n108 = Reverse 1D Array(array=w208) -> (reversed array=w194:i32[])
        n109 = Array Size(array=w195) -> (size(s)=w206:i32)
        n110 = for {
          tunnel: w194 -> [w241] mode=indexing
          tunnel: w207 -> [w243]
          shift-right: [w244] -> w198
          shift-left: w207 -> [w245]
          i -> [w242]
          n111 = Index Array(array=w243, index (col)=w241) -> (element=w240:dbl[])  [unwired: 1 in]
          n112 = Replace Array Subset(array=w245, new element=w240, index (col)=w242) -> (w244:dbl[][])  [unwired: 1 in]
        }
        "eVec" <- w198
        n113 = for {
          N: 2 -> [_]
          tunnel: w200 -> [w235]
          tunnel: w198 -> [w239]
          tunnel: [w230] -> w196 mode=indexing
          tunnel: [w229] -> w197 mode=indexing
          i -> [w238]
          n114 = Index Array(array=w239, index (col)=w238) -> (element=w237:dbl[])  [unwired: 1 in]
          n115 = call-poly <vilib>:"Array To Matrix.vi"("Real 1D Array"=w237) -> ("Real Matrix (Column Vector)"=w236:T7)
          n116 = call-poly <vilib>:"Multiply.vi"("Real Matrix B"=w236, "Real Matrix A"=w235) -> ("A * B"=w234:T7)
          n117 = call-poly <vilib>:"Matrix To Array.vi"("Real Matrix"=w234) -> ("Real 2D Array"=w233:dbl[][])
          n118 = Index Array(array=w233, index (col)=0 ("disabled index (col)")) -> (element=w231:dbl[])  [unwired: 1 in]
          n119 = Decimate 1D Array(w231) -> (w230:dbl[], w229:dbl[])
        }
        n120 = Decrement(x=w206) -> (x-1=w204:i32)
        n121 = in-place {
          n122 = in-place-array #3(w195, w204) -> ()  [unwired: 1 out]
          n123 = in-place-array #3(0.0 ("element")) -> (w203:dbl[])  [unwired: 1 out]
        }
        "eVal" <- w203
        n124 = Transpose 2D Array(2D array=w197) -> (transposed array=→"v(Spot,mode)":dbl[][])
        n125 = Transpose 2D Array(2D array=w196) -> (transposed array=→"u(Spot,mode)":dbl[][])
        n126 = Add Array Elements(numeric array=w203) -> (sum=w202:dbl)
        n127 = Divide(x=w203, y=w202) -> (x/y=→"Modal Energy":dbl[])
      }
      frame "Create Files" {
        n128 = Index Array(array=w302) -> (element=w314:T3)  [unwired: 1 in]
        n129 = Equal?(x=w298, y=1) -> (x = y?=w293:bool)
        n130 = Build Path(base path=w316, name or relative path=w317) -> (appended path=w296:path)
        n131 = call "Get Cluster Element Names.vi"("Cluster"=w314) -> ("Element Names"=w313:string[])  [unwired: 9 in, 1 out]
        n132 = Unbundle By Name(w314) -> ("Turb Stats"=w304:T5)
        n133 = call <vilib>:"Check if File or Folder Exists.vi"("path"=w296) -> ("file or folder exists?"=w294:bool, "dup path"=w295:path)  [unwired: 8 in, 1 out]
        n134 = And(x=w293, y=w294) -> (x .and. y?=w290:bool)
        n135 = case shown="True" w290 {
          tunnel: [w325 path "" ("dup path")] -> w282
          tunnel: w295 -> [w325 _]
          frame False {
          }
          frame True {
            w328 = T9 1 items=["no dialog", "OK message", "continue or stop message", "OK message + warnings", "continue/stop + warnings"] ("type of dialog (OK msg:1)")
            n136 = call <vilib>:"Simple Error Handler.vi"("type of dialog (OK msg:1)"=w328, "error in (no error)"=errorcluster {"status"=TRUE, "code"=0, "source"="Folder already exists, please select a new case name or results folder"}) -> ()  [unwired: 3 in, 5 out]
          }
        }
        n137 = Delete From Array(array=w313, length=10, index=1) -> (deleted portion=w301:string[], array with subset deleted=w309:string[])
        n138 = Index Array(array=w304) -> (element=w303:T4)  [unwired: 1 in]
        n139 = call "Get Cluster Element Names.vi"("Cluster"=w303) -> ("Element Names"=w310:string[])  [unwired: 9 in, 1 out]
        n140 = Delete From Array(array=w301, length=2, index=6) -> (deleted portion=w279:string[])  [unwired: 1 out]
        n141 = for {
          tunnel: w279 -> [w331] mode=indexing
          tunnel: w310 -> [w330]
          tunnel: [w329] -> w308 mode=indexing
          n142 = for {
            tunnel: w331 -> [w335]
            tunnel: w330 -> [w333] mode=indexing
            tunnel: [w332] -> w329 mode=indexing
            n143 = Concatenate Strings(w335, "_" ("string"), w333) -> (w332:string)
          }
        }
        n144 = Index Array(array=w308) -> (element #1=w307:string[], element #2=w306:string[])  [unwired: 4 in]
        n145 = Build Array (concatenate)(w309, w307, w306) -> (w305:string[])
        n146 = for {
          tunnel: w305 -> [w338] mode=indexing
          tunnel: [w340] -> w283 mode=indexing
          w344 = "_" ("Replace with")
          n147 = call <vilib>:"Trim Whitespace.vi"("string"=w338) -> ("trimmed string"=w336:string)  [unwired: 1 in]
          n148 = call "Replace_Character.vi"("Replace with"="_", "Input String"=w336, "Search For"=" ") -> ("Output string"=w339:string)  [unwired: 1 out]
          n149 = call "Replace_Character.vi"("Replace with"=w344, "Input String"=w339, "Search For"="(") -> ("Output string"=w346:string)  [unwired: 1 out]
          n150 = call "Replace_Character.vi"("Replace with"=w344, "Input String"=w346, "Search For"=")") -> ("Output string"=w343:string)  [unwired: 1 out]
          n151 = call "Replace_Character.vi"("Replace with"="", "Input String"=w343, "Search For"="/") -> ("Output string"=w340:string)  [unwired: 1 out]
        }
        "Variable Names" <- w283
        n152 = for {
          tunnel: w282 -> [w324]
          tunnel: [w318] -> w288 mode=indexing
          tunnel: w283 -> [_] mode=indexing
          i -> [w323]
          n153 = Increment(x=w323) -> (x+1=w322:i32)
          n154 = Number To Decimal String(number=w322) -> (decimal integer string=w320:string)  [unwired: 1 in]
          n155 = Concatenate Strings("ENSI.var" ("name or relative path"), w320) -> (w319:string)
          n156 = Build Path(base path=w324, name or relative path=w319) -> (appended path=w318:path)
        }
        n157 = Build Path(base path=w282, name or relative path="ENSI.case") -> (appended path=w286:path)
        n158 = Build Path(base path=w282, name or relative path="ENSI.geo") -> (appended path=w287:path)
        n159 = Build Array (concatenate)(w286, w287, w288) -> (→"File Paths":path[])
        n160 = Select(t="End Time", s=w290, f="Setup Files" ("t")) -> (s? t:f=w292:string)
      }
      frame "Setup Files" {
        n161 = local read "File Paths"() -> (w354:path[])
        n162 = local write "Status"("Setting up case files ready to write to..." ("Status")) -> ()
        n163 = for {
          N -> [w357]
          tunnel: w354 -> [w360] mode=indexing
          i -> [w355]
          n164 = Divide(x=w355, y=w357) -> (x/y=w356:dbl)
          n165 = Multiply(x=w356, y=100) -> (x*y=w359:dbl)
          n166 = local write "Progress Bar"(w359) -> ()
          n167 = case shown="0" w355 {
            tunnel: w360 -> [w365 w386 w405]
            tunnel: w355 -> [_ _ w400]
            frame 0 {
              n168 = local read "Variable Names"() -> (w362:string[])
              n169 = for {
                tunnel: w362 -> [w371] mode=indexing
                tunnel: [w369] -> w361 mode=indexing
                i -> [w374]
                n170 = Increment(x=w374) -> (x+1=w375:i32)
                n171 = Number To Decimal String(number=w375) -> (decimal integer string=w372:string)  [unwired: 1 in]
                n172 = Concatenate Strings(" ENSI.var", w372) -> (w370:string)
                n173 = Concatenate Strings("scalar per node: ", w371, w370) -> (w369:string)
              }
              n174 = Build Array (concatenate)(string[] ["FORMAT", "type: ensight gold", "GEOMETRY", "model: ENSI.geo", "VARIABLE"], w361) -> (w364:string[])
              n175 = for {
                tunnel: w364 -> [w381] mode=indexing
                shift-right: [w379] -> w367
                shift-left: "" -> [w377]
                n176 = Concatenate Strings(w381, "\n") -> (w378:string)
                n177 = Concatenate Strings(w377, w378) -> (w379:string)
              }
              n178 = call "Write_File_Simple.vi"("append to file? (new file:F)"=FALSE, "character string"=w367, "file path"=w365) -> ()  [unwired: 2 out]
            }
            frame 1 {
              n179 = local read "# total vectors"() -> (w384:i32)
              n180 = Number To Decimal String(number=w384) -> (decimal integer string=w383:string)  [unwired: 1 in]
              n181 = Build Array (concatenate)(string[] ["EnSight Model Geometry File", "EnSight 9.2 ", "node id assign", "element id assign", "part", "         1", "Point field", "coordinates"], w383) -> (w382:string[])
              n182 = for {
                tunnel: w382 -> [w394] mode=indexing
                shift-right: [w392] -> w388
                shift-left: "" -> [w390]
                n183 = Concatenate Strings(w394, "\n") -> (w391:string)
                n184 = Concatenate Strings(w390, w391) -> (w392:string)
              }
              n185 = call "Write_File_Simple.vi"("append to file? (new file:F)"=FALSE, "character string"=w388, "file path"=w386) -> ()  [unwired: 2 out]
            }
            frame 2, Default {
              n186 = local read "Variable Names"() -> (w401:string[])
              n187 = Subtract(x=w400, y=2) -> (x-y=w398:i32)
              n188 = Index Array(array=w401, index=w398) -> (element=w397:string)
              n189 = Build Array (concatenate)(w397, string[] ["part", "         1", "coordinates"]) -> (w395:string[])
              n190 = for {
                tunnel: w395 -> [w410] mode=indexing
                shift-right: [w408] -> w403
                shift-left: "" -> [w406]
                n191 = Concatenate Strings(w410, "\n") -> (w407:string)
                n192 = Concatenate Strings(w406, w407) -> (w408:string)
              }
              n193 = call "Write_File_Simple.vi"("append to file? (new file:F)"=FALSE, "character string"=w403, "file path"=w405) -> ()  [unwired: 2 out]
            }
          }
        }
      }
      frame "Collect Data" {
        w415 = T6 []  # Array
        n194 = for {
          N -> [w426]
          tunnel: w417 -> [w434] mode=indexing
          tunnel: [w432] -> w411 mode=indexing
          tunnel: [w431] -> w413 mode=indexing
          i -> [w427]
          n195 = Unbundle By Name(w434) -> ("Record Length"=w433:dbl, "Turb Stats"=w425:T5, "Turb Stats Error"=w422:T5, "XYZ Position"=w431:dbl[])
          n196 = Divide(x=w427, y=w426) -> (x/y=w429:dbl)
          n197 = Multiply(x=w429, y=100) -> (x*y=w430:dbl)
          n198 = local write "Progress Bar"(w430) -> ()
          n199 = Index Array(array=w425) -> (element=w424:T4)  [unwired: 1 in]
          n200 = Index Array(array=w422) -> (element=w421:T4)  [unwired: 1 in]
          n201 = Cluster To Array(cluster=w424) -> (array=w423:dbl[])
          n202 = Cluster To Array(cluster=w421) -> (array=w420:dbl[])
          n203 = Build Array (concatenate)(w433, w423, w420) -> (w432:dbl[])
        }
        "Data Array (spot,Var)" <- w411
        n204 = local write "Status"("Gathering all the data ready to write to file..." ("Status")) -> ()
        n205 = Transpose 2D Array(2D array=w413) -> (transposed array=→"Position Array (XYZ,spot)":dbl[][])
      }
      frame "Save Data" {
        n206 = local read "Data Array (spot,Var)"() -> (w439:dbl[][])
        n207 = local read "Position Array (XYZ,spot)"() -> (w438:dbl[][])
        n208 = local read "File Paths"() -> (w440:path[])
        n209 = Transpose 2D Array(2D array=w439) -> (transposed array=w435:dbl[][])
        n210 = local write "Status"("Wrting the data to file..." ("Status")) -> ()
        n211 = for {
          N -> [w444]
          tunnel: w440 -> [w451] mode=indexing
          tunnel: w435 -> [w450]
          tunnel: w438 -> [w449]
          i -> [w445]
          # "Loop Variable"
          n212 = Divide(x=w445, y=w444) -> (x/y=w447:dbl)
          n213 = Multiply(x=w447, y=100) -> (x*y=w448:dbl)
          n214 = local write "Progress Bar"(w448) -> ()
          n215 = case shown="2, Default" w445 {
            tunnel: w451 -> [_ w457 w469]
            tunnel: w445 -> [_ _ w476]
            tunnel: w450 -> [_ _ w473]
            tunnel: w449 -> [_ w456 _]
            frame 0 {
            }
            frame 1 {
              n216 = Index Array(array=w456) -> (element #1=w455:dbl[], element #2=w454:dbl[], element #3=w453:dbl[])  [unwired: 6 in]
              n217 = Build Array (concatenate)(w455, w454, w453) -> (w452:dbl[])
              n218 = for {
                tunnel: w452 -> [w461] mode=indexing
                shift-right: [w467] -> w458
                shift-left: "" -> [w466]
                w462 = T9 4 items=["no dialog", "OK message", "continue or stop message", "OK message + warnings", "continue/stop + warnings"] ("type of dialog (OK msg:1)")
                n219 = call "Ensight_Format_Check.vi"("Input Number"=w461) -> ("error"=w464:errorcluster, "Output string"=w465:string)  [unwired: 8 in, 1 out]
                n220 = Concatenate Strings(w466, w465) -> (w467:string)
                n221 = call <vilib>:"Simple Error Handler.vi"("error source (\" \")"="GEOM" ("error source (\" \")"), "type of dialog (OK msg:1)"=w462, "error in (no error)"=w464) -> ()  [unwired: 2 in, 5 out]
              }
              n222 = call "Write_File_Simple.vi"("append to file? (new file:F)"=TRUE, "character string"=w458, "file path"=w457) -> ()  [unwired: 2 out]
            }
            frame 2, Default {
              n223 = Subtract(x=w476, y=2) -> (x-y=w468:i32)
              n224 = Index Array(array=w473, index (row)=w468) -> (element=w472:dbl[])  [unwired: 1 in]
              n225 = for {
                tunnel: w472 -> [w477] mode=indexing
                shift-right: [w486] -> w470
                shift-left: "" -> [w485]
                tunnel: w469 -> [w482]
                w478 = T9 4 items=["no dialog", "OK message", "continue or stop message", "OK message + warnings", "continue/stop + warnings"] ("type of dialog (OK msg:1)")
                n226 = Path To String(path=w482) -> (string=w481:string)
                n227 = call "Ensight_Format_Check.vi"("Input Number"=w477) -> ("error"=w483:errorcluster, "Output string"=w484:string)  [unwired: 8 in, 1 out]
                n228 = Concatenate Strings("VAR file: " ("error source (\" \")"), w481) -> (w479:string)
                n229 = call <vilib>:"Simple Error Handler.vi"("error source (\" \")"=w479, "type of dialog (OK msg:1)"=w478, "error in (no error)"=w483) -> ()  [unwired: 2 in, 5 out]
                n230 = Concatenate Strings(w485, w484) -> (w486:string)
              }
              n231 = call "Write_File_Simple.vi"("append to file? (new file:F)"=TRUE, "character string"=w470, "file path"=w469) -> ()  [unwired: 2 out]
            }
          }
        }
      }
      frame "End Time" {
        n232 = local write "Position Array (XYZ,spot)"(dbl[][] [] ("Position Array")) -> ()
        n233 = local write "Data Array (spot,Var)"(dbl[][] [] ("Data Array")) -> ()
      }
    }
  }
  "Progress Bar" <- u8 0 ("Progress Bar")
